vi "Multiple USB Camera Acquisition 2009.vi"() -> ()   [LabVIEW 2016]
uses:
  <vilib>/userdefined/High Color/IMAQdx.ctl
  <vilib>/vision/driver/NI_Vision_Acquisition_Software.lvlib
panel:
  in  "Stop":bool
  out "Image":T1(plugin-control)
  in  "Camera Name":T2
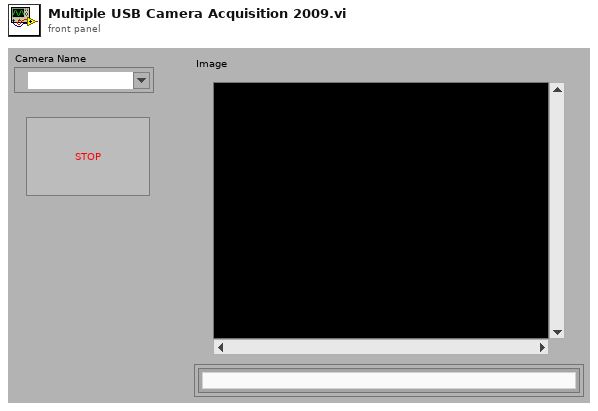
[diagram p1: front panel]
types:
  T1 = typedef "IMAQ Image.ctl" = refnum<image>
  T2 = typedef "IMAQdx.ctl" = refnum<k21>
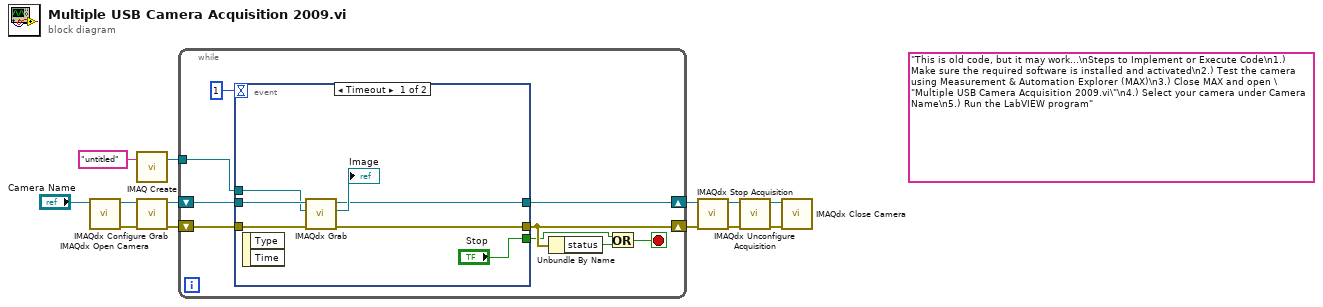
[diagram p0: block diagram]
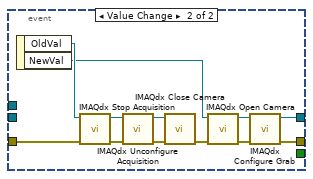
[diagram p2: hidden frame]
diagram:
  (unwired) "This is old code, but it may work...\nSteps to Implement or Execute Code\n1.) Make sure the required software is installed and activated\n2.) Test the camera using Measurement & Automation Explorer (MAX)\n3.) Close MAX and open \"Multiple USB Camera Acquisition 2009.vi\"\n4.) Select your camera under Camera Name\n5.) Run the LabVIEW program"
  n1 = call <vilib>:"IMAQdx Open Camera.vi"("Session In"="Camera Name") -> ("error out"=w3:errorcluster, "Session Out"=w8:T2)  [unwired: 2 in, 7 out]
  n2 = call "IMAQ Create"("Image Name"="untitled") -> ("New Image"=w4:T1)  [unwired: 3 in, 2 out]
  n3 = call <vilib>:"IMAQdx Configure Grab.vi"("error in"=w3, "Session In"=w8) -> ("error out"=w2:errorcluster, "Session Out"=w7:T2)  [unwired: 8 in]
  n4 = while {
    shift-right: [w21] -> w9
    shift-left: w7 -> [w20]
    tunnel: w4 -> [w19]
    shift-right: [w17] -> w1
    shift-left: w2 -> [w18]
    stop <- w14 stop-if-true
    n5 = event shown="[0] Timeout" {
      selector: _ -> [_ _]
      dyn-events: _ -> [_ _]
      timeout: 1 -> [_ _]
      tunnel: [w27 w39] -> w21
      tunnel: ["Stop" _] -> w15
      tunnel: w20 -> [w26 _]
      tunnel: w19 -> [w25 _]
      tunnel: w18 -> [w24 w31]
      tunnel: [w23 w30] -> w17
      event Timeout {
        n6 = event-data() -> ()  [unwired: 1 in, 2 out]
        n7 = call <vilib>:"IMAQdx Grab.vi"("error in"=w24, "Image In"=w25, "Session In"=w26) -> ("error out"=w23:errorcluster, "Image Out"=→"Image":T1, "Session Out"=w27:T2)  [unwired: 5 in, 1 out]
      }
      event Value Change {
        n8 = event-data() -> ("OldVal"=w41:T2, "NewVal"=w36:T2)  [unwired: 1 in]
        n9 = call <vilib>:"IMAQdx Stop Acquisition.vi"("error in"=w31, "Session In"=w41) -> ("error out"=w32:errorcluster, "Session Out"=w33:T2)  [unwired: 8 out]
        n10 = call <vilib>:"IMAQdx Unconfigure Acquisition.vi"("error in"=w32, "Session In"=w33) -> ("error out"=w35:errorcluster, "Session Out"=w34:T2)  [unwired: 8 out]
        n11 = call <vilib>:"IMAQdx Close Camera.vi"("error in"=w35, "Session In"=w34) -> ("error out"=w38:errorcluster)  [unwired: 9 out]
        n12 = call <vilib>:"IMAQdx Open Camera.vi"("error in"=w38, "Session In"=w36) -> ("error out"=w37:errorcluster, "Session Out"=w40:T2)  [unwired: 1 in, 7 out]
        n13 = call <vilib>:"IMAQdx Configure Grab.vi"("error in"=w37, "Session In"=w40) -> ("error out"=w30:errorcluster, "Session Out"=w39:T2)  [unwired: 8 in]
      }
    }
    n14 = Unbundle By Name(w17) -> ("status"=w16:bool)
    n15 = Or(x=w15, y=w16) -> (x .or. y?=w14:bool)
  }
  n16 = call <vilib>:"IMAQdx Stop Acquisition.vi"("error in"=w1, "Session In"=w9) -> ("error out"=w10:errorcluster, "Session Out"=w11:T2)  [unwired: 8 out]
  n17 = call <vilib>:"IMAQdx Unconfigure Acquisition.vi"("error in"=w10, "Session In"=w11) -> ("error out"=w13:errorcluster, "Session Out"=w12:T2)  [unwired: 8 out]
  n18 = call <vilib>:"IMAQdx Close Camera.vi"("error in"=w13, "Session In"=w12) -> ()  [unwired: 10 out]
